vi "7.vi"() -> ()   [LabVIEW 2017]
panel:
  out "波形图表":cluster{dbl, "y":dbl, "y":dbl}(graph)
  in  "停止":bool
  out "高温":bool
  out "低温":bool
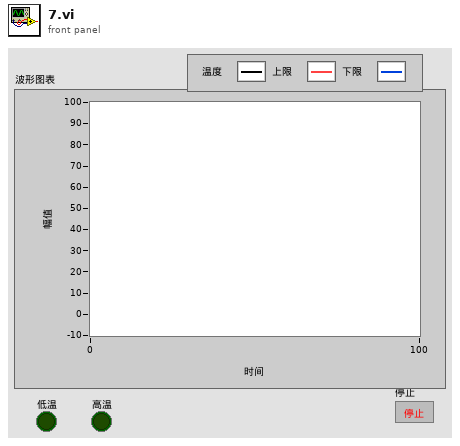
[diagram p1: front panel]
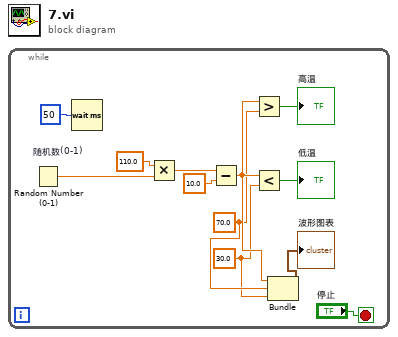
[diagram p0: block diagram]
diagram:
  n1 = while {
    stop <- "停止" stop-if-true
    w2 = 30.0 ("y")
    w3 = 70.0 ("y")
    n2 = Random Number (0-1) "随机数(0-1)"() -> (number: 0 to 1=w11:dbl)
    n3 = Wait (ms)(milliseconds to wait=u32 50 ("等待时间（毫秒）")) -> ()  [unwired: 1 out]
    n4 = Multiply(x=110.0, y=w11) -> (x*y=w9:dbl)
    n5 = Subtract(x=w9, y=10.0) -> (x-y=w4:dbl)
    n6 = Greater?(x=w4, y=w3) -> (0:→"高温":bool)
    n7 = Less?(x=w4, y=w2) -> (x < y?=→"低温":bool)
    n8 = Bundle(w4, "y"=w3, "y"=w2) -> (→"波形图表":cluster{dbl, "y":dbl, "y":dbl})  [unwired: 1 in]
  }
